vi "Unflatten.vi"(8 "error in (no error)":errorcluster, 10 "JSON stream":string, 11 "JSON Array in":refnum<class "JSON Array.lvclass">) -> (0 "error out":errorcluster, 1 "Empty?":bool, 2 "rest of JSON stream":string, 3 "JSON Array out":refnum<class "JSON Array.lvclass">)   [LabVIEW 2020, in "Library Commun.lvlib" / "JSON Array.lvclass"]
uses:
  JSON Array.lvclass
  JSON Value/JSON Value.lvclass
  JSON Array.lvclass/JSON Array.ctl
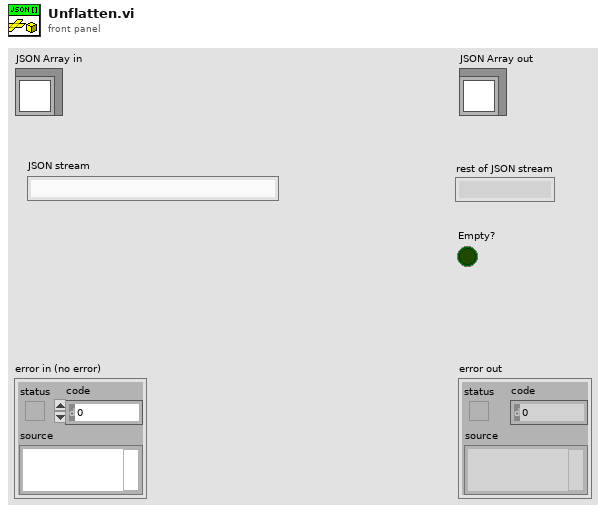
[diagram p1: front panel]
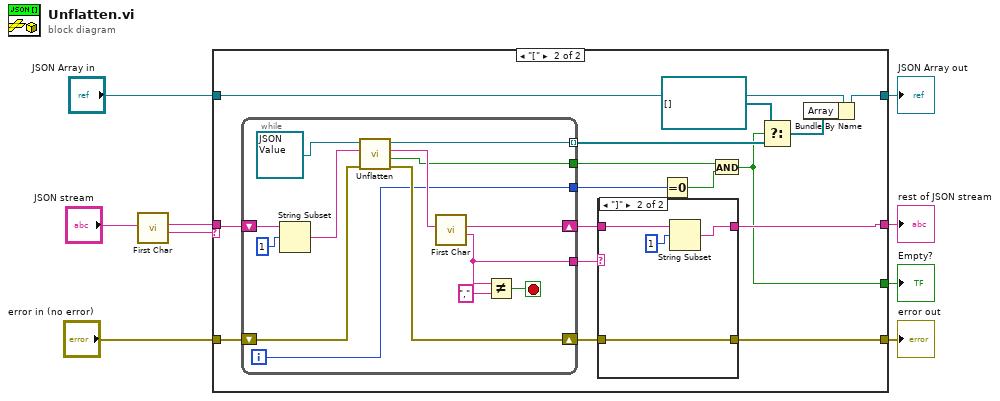
[diagram p0: block diagram]
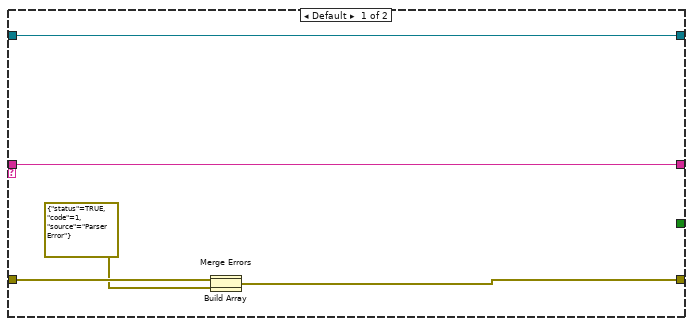
[diagram p2: hidden frame]
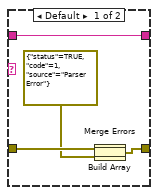
[diagram p3: hidden frame]
diagram:
  n1 = call "First Char.vi"("String in"="JSON stream") -> ("First Char"=w8:string, "String"=w7:string)  [unwired: 9 in]
  n2 = case shown="\"[\"" w8 {
    tunnel: w7 -> [w12 w31]
    tunnel: [w14 w24] -> w6
    tunnel: "error in (no error)" -> [w15 w28]
    tunnel: [w12 w26] -> w4
    tunnel: [w11 w29] -> w3
    tunnel: "JSON Array in" -> [w11 w30]
    tunnel: [_ w16] -> w1
    frame Default {
      n3 = Build Array(w15, errorcluster {"status"=TRUE, "code"=1, "source"="Parser Error"} ("error in")) -> (w10:errorcluster[])
      n4 = Merge Errors(w10) -> (w14:errorcluster)
    }
    frame "[" {
      n5 = while {
        shift-right: [w48] -> w27
        shift-left: w31 -> [w53]
        tunnel: [w47] -> w18 mode=indexing
        tunnel: [w46] -> w25
        shift-right: [w44] -> w23
        shift-left: w28 -> [w45]
        tunnel: [w42] -> w21
        tunnel: [w41] -> w20
        i -> [w41]
        stop <- w49 stop-if-true
        n6 = String Subset(string=w53, offset (0)=1 ("length (rest)")) -> (substring=w52:string)  [unwired: 1 in]
        n7 = call-dynamic "Unflatten.vi"("error in (no error)"=w45, "JSON stream"=w52, "JSON Value in"=refnum<class "JSON Value.lvclass"> refnum ("JSON Value.lvclass")) -> ("error out"=w44:errorcluster, "Empty?"=w42:bool, "rest of JSON stream"=w51:string, "JSON Value out"=w47:refnum<class "JSON Value.lvclass">)  [unwired: 5 in]
        n8 = call "First Char.vi"("String in"=w51) -> ("First Char"=w46:string, "String"=w48:string)  [unwired: 9 in]
        n9 = Not Equal?(x=w46, y=",") -> (x != y?=w49:bool)
      }
      n10 = case shown="\"]\"" w25 {
        tunnel: w27 -> [w33 w39]
        tunnel: [w33 w38] -> w26
        tunnel: [w35 w37] -> w24
        tunnel: w23 -> [w36 w37]
        frame Default {
          n11 = Build Array(w36, errorcluster {"status"=TRUE, "code"=1, "source"="Parser Error"} ("error in")) -> (w32:errorcluster[])
          n12 = Merge Errors(w32) -> (w35:errorcluster)
        }
        frame "]" {
          n13 = String Subset(string=w39, offset (0)=1 ("length (rest)")) -> (substring=w38:string)  [unwired: 1 in]
        }
      }
      n14 = Equal To 0?(x=w20) -> (x = 0?=w22:bool)
      n15 = And(x=w21, y=w22) -> (x .and. y?=w16:bool)
      n16 = Select(t=refnum<class "JSON Value.lvclass">[] [], s=w16, f=w18) -> (s? t:f=w19:refnum<class "JSON Value.lvclass">[])
      n17 = Bundle By Name(cluster=w30, "Array"=w19) -> (w29:refnum<class "JSON Array.lvclass">)
    }
  }
  "error out" <- w6
  "JSON Array out" <- w3
  "rest of JSON stream" <- w4
  "Empty?" <- w1
